vi "System@UserPanelOpen__Parameter.vi"(1 "ParamterIn":string) -> (0 "ParamterOut":string)   [LabVIEW 2020]
uses:
  MainFrame/Global.vi
panel:
  in  "Parameters":string(combo)
  in  "VI":string(combo)
  in  "Confirm":bool
  # "System@UserPanelOpen $VI,$Parameter\nSystem@UserPanelOpen DynamicPanel,$Panel.DynPnl\nSystem@UserPanelOpen  --> Close UserPanel"
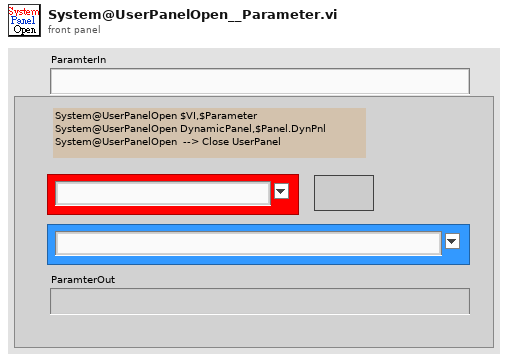
[diagram p1: front panel]
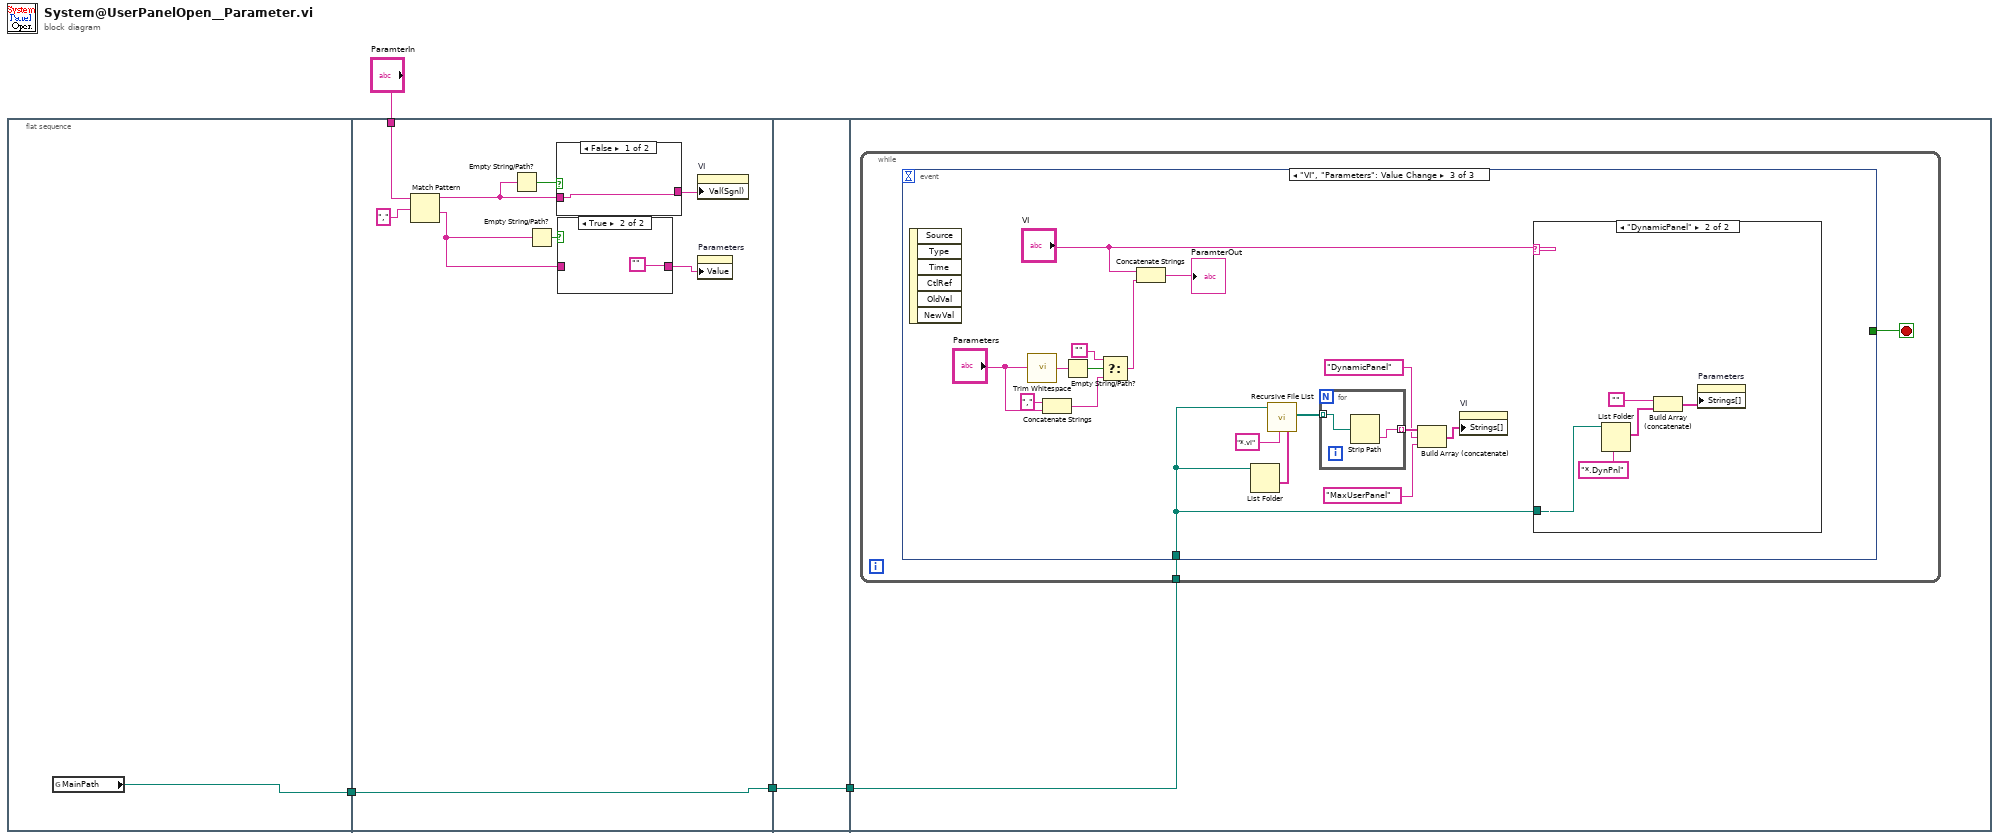
[diagram p0: block diagram]
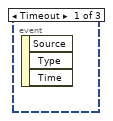
[diagram p4: hidden frame]
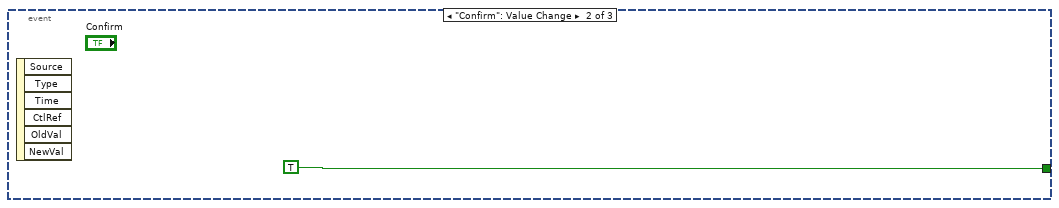
[diagram p5: hidden frame]
diagram:
  n1 = flat-sequence {
    tunnel: [w5] -> w1
    tunnel: "ParamterIn" -> [w11]
    tunnel: [w12] -> w2
    tunnel: w1 -> [w12]
    tunnel: [w19] -> w3
    tunnel: w2 -> [w19]
    tunnel: w3 -> [w20]
    frame #0 {
      n2 = global read "Global.vi" "MainPath"() -> (w5:path)
    }
    frame #1 {
      n3 = Match Pattern(string=w11, regular expression=",") -> (before substring=w9:string, after substring=w8:string)  [unwired: 1 in, 2 out]
      n4 = Empty String/Path?(string/path=w9) -> (empty?=w14:bool)
      n5 = Empty String/Path?(string/path=w8) -> (empty?=w13:bool)
      n6 = case shown="False" w14 {
        tunnel: w9 -> [w17 w18]
        tunnel: [w17 w18] -> w6
        frame False {
        }
        frame True {
        }
      }
      n7 = case shown="True" w13 {
        tunnel: [w15 ""] -> w7
        tunnel: w8 -> [w15 _]
        frame False {
        }
        frame True {
        }
      }
      n8 = property on="VI" class="CmbBox"("Val(Sgnl)"=w6) -> ()  [unwired: 2 in, 2 out]
      n9 = property on="Parameters" class="CmbBox"("Value"=w7) -> ()  [unwired: 2 in, 2 out]
    }
    frame #2 {
    }
    frame #3 {
      n10 = while {
        tunnel: w20 -> [w21]
        stop <- w22 stop-if-true
        n11 = event shown="[2] \"VI\", \"Parameters\": Value Change" {
          selector: _ -> [_ _ _]
          dyn-events: _ -> [_ _ _]
          timeout: _ -> [_ _ _]
          tunnel: [_ TRUE _] -> w22
          tunnel: w21 -> [_ _ w26]
          event Timeout {
            n12 = event-data() -> ()  [unwired: 1 in, 3 out]
          }
          event "Confirm": Value Change {
            n13 = event-data() -> ()  [unwired: 1 in, 6 out]
          }
          event "VI", "Parameters": Value Change {
            n14 = event-data() -> ()  [unwired: 1 in, 6 out]
            n15 = call <vilib>:"Trim Whitespace.vi"("string"="Parameters") -> ("trimmed string"=w35:string)  [unwired: 1 in]
            n16 = Concatenate Strings("," ("string"), "Parameters") -> (w34:string)
            n17 = Empty String/Path?(string/path=w35) -> (empty?=w36:bool)
            n18 = Select(t="", s=w36, f=w34) -> (s? t:f=w31:string)
            n19 = Concatenate Strings("VI", w31) -> (→"ParamterOut":string)
            n20 = List Folder(path=w26) -> (folder names=w30:string[])  [unwired: 3 in, 3 out]
            n21 = call <vilib>:"Recursive File List.vi"("Folders to Exclude"=w30, "pattern"="*.vi", "Folder Path"=w26) -> ("All Files in Dir"=w39:path[])  [unwired: 4 in, 4 out]
            n22 = for {
              tunnel: w39 -> [w47] mode=indexing
              tunnel: [w46] -> w29 mode=indexing
              n23 = Strip Path(path=w47) -> (name=w46:string)  [unwired: 1 out]
            }
            n24 = Build Array (concatenate)(w29, "DynamicPanel", "MaxUserPanel") -> (w28:string[])
            n25 = property on="VI" class="CmbBox"("Strings[]"=w28) -> ()  [unwired: 2 in, 2 out]
            n26 = case shown="\"DynamicPanel\"" "VI" {
              tunnel: w26 -> [_ w45]
              frame "False", Default {
              }
              frame "DynamicPanel" {
                n27 = List Folder(path=w45, pattern="*.DynPnl") -> (filenames=w43:string[])  [unwired: 2 in, 3 out]
                n28 = Build Array (concatenate)("", w43) -> (w41:string[])
                n29 = property on="Parameters" class="CmbBox"("Strings[]"=w41) -> ()  [unwired: 2 in, 2 out]
              }
            }
          }
        }
      }
    }
  }
